vi "SUPPORT.vi"() -> ()   [LabVIEW 2016, in "update.lvlib"]
uses:
  update.lvlib
panel:
  out "msg":string
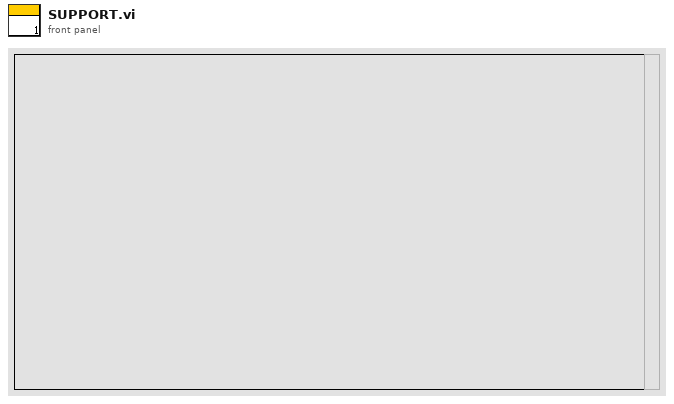
[diagram p1: front panel]
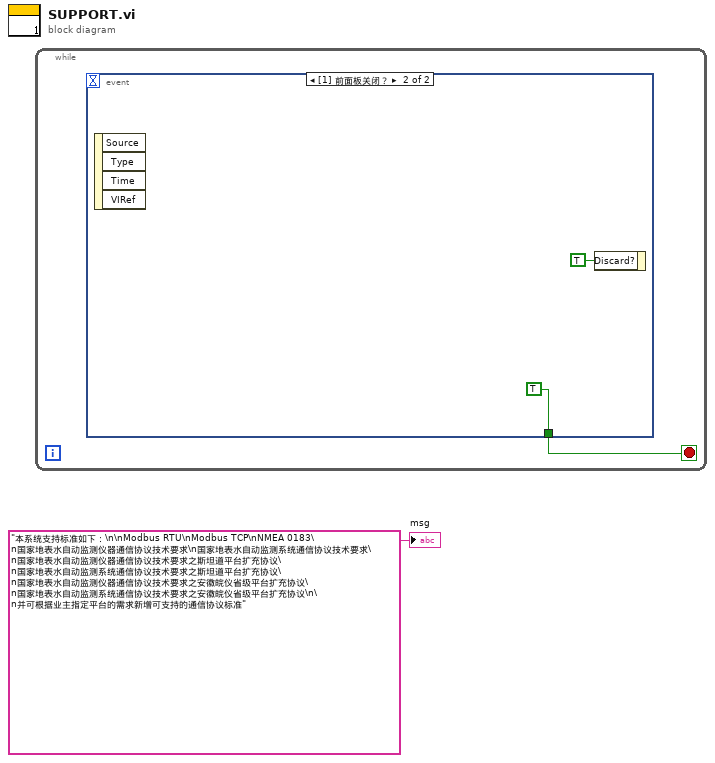
[diagram p0: block diagram]
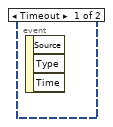
[diagram p2: hidden frame]
diagram:
  n1 = while {
    stop <- w2 stop-if-true
    n2 = event shown="[1] 前面板关闭？" {
      selector: _ -> [_ _]
      dyn-events: _ -> [_ _]
      timeout: _ -> [_ _]
      tunnel: [_ TRUE] -> w2
      event Timeout {
        n3 = event-data() -> ()  [unwired: 1 in, 3 out]
      }
      event Panel Close? {
        n4 = event-data() -> ()  [unwired: 1 in, 4 out]
        n5 = event-data("Discard?"=TRUE ("放弃？")) -> ()  [unwired: 1 in, 1 out]
      }
    }
  }
  "msg" <- "本系统支持标准如下：\n\nModbus RTU\nModbus TCP\nNMEA 0183\n国家地表水自动监测仪器通信协议技术要求\n国家地表水自动监测系统通信协议技术要求\n国家地表水自动监测仪器通信协议技术要求之斯坦道平台扩充协议\n国家地表水自动监测系统通信协议技术要求之斯坦道平台扩充协议\n国家地表水自动监测仪器通信协议技术要求之安徽皖仪省级平台扩充协议\n国家地表水自动监测系统通信协议技术要求之安徽皖仪省级平台扩充协议\n\n并可根据业主指定平台的需求新增可支持的通信协议标准" ("msg")
